vi "Enable TLAST.vi"(10 "s_axis_tlast":refnum<k21>, 11 "niInstr AXI4-Stream Writer v1 FPGA in":refnum<class "niInstr AXI4-Stream Writer v1 FPGA.lvclass">) -> (3 "niInstr AXI4-Stream Writer v1 FPGA out":refnum<class "niInstr AXI4-Stream Writer v1 FPGA.lvclass">)   [LabVIEW 2015, in "niInstr AXI4-Stream Writer v1 FPGA.lvclass"]
doc: "Enables TLAST to be compiled in as part of the AXI4-Stream Writer interface.\n\n<B>Input Parameters</B>\n\n<B>s_axis_tlast</B> is the FPGA resource to use for TLAST.\n\n<B>niInstr AXI4-Stream Writer v1 FPGA in</B> takes in a reference to the AXI4-Stream Writer from the previous VI.\n\n<B>Output Parameters</B>\n\n<B>niInstr AXI4-Stream Writer v1 FPGA out</B> passes a reference to the AXI4-Stream Writer to the next VI."
uses:
  <instrlib>/_niInstr/CLIP Adapters/v1/FPGA/AXI4-Stream/Writer/niInstr AXI4-Stream Writer v1 FPGA.lvclass
  <instrlib>/_niInstr/CLIP Adapters/v1/FPGA/AXI4-Stream/Writer/niInstr AXI4-Stream Writer v1 FPGA.lvclass/niInstr AXI4-Stream Writer v1 FPGA.ctl
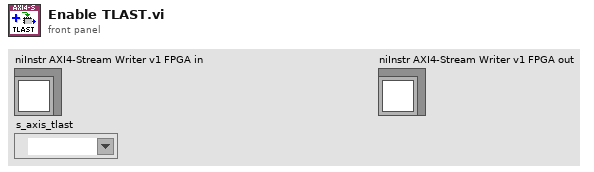
[diagram p1: front panel]
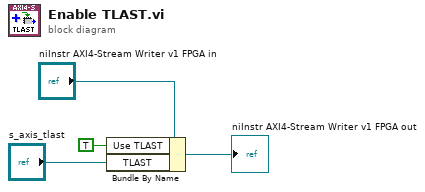
[diagram p0: block diagram]
diagram:
  n1 = Bundle By Name(cluster="niInstr AXI4-Stream Writer v1 FPGA in", "Use TLAST"=TRUE ("Use TREADY"), "TLAST"="s_axis_tlast") -> (→"niInstr AXI4-Stream Writer v1 FPGA out":refnum<class "niInstr AXI4-Stream Writer v1 FPGA.lvclass">)
